vi "Protection and Rolling Counter Addon SysDef Example.vi"() -> (0 "error out":errorcluster)   [LabVIEW 2025]
uses:
  NationalInstruments.VeriStand.Internal
  NationalInstruments.VeriStand.SystemDefinitionAPI
  Protection and Counter Addon System Definition API.lvlib
panel:
  in  "Configuration (.dat)":path
  in  "error in (no error)":errorcluster
  out "Sysdef Path":path=path "C:/Users/Public/Documents/National Instruments/NI VeriStand 2013/DynamicallyCreatedProject/DynamicallyCreatedProject.nivssdf"
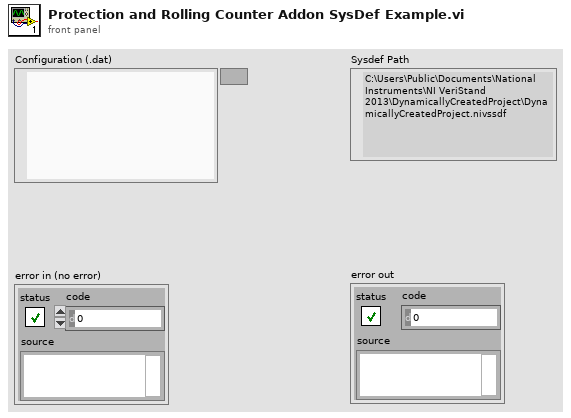
[diagram p1: front panel]
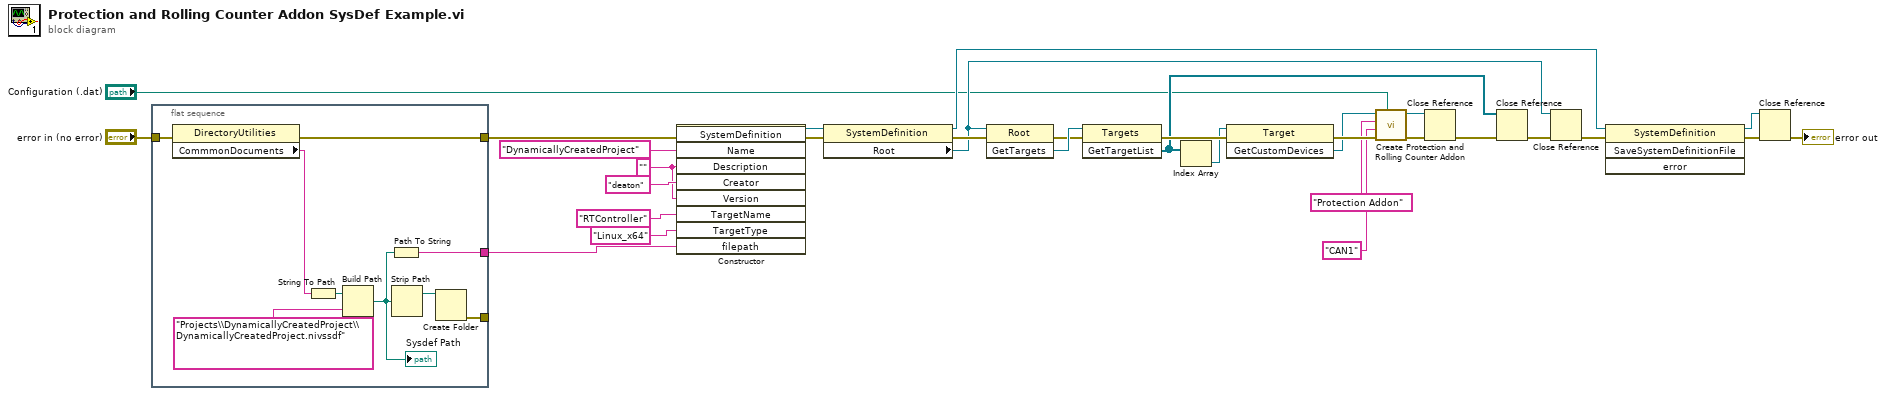
[diagram p0: block diagram]
diagram:
  w28 = "" ("Description")
  n1 = flat-sequence {
    tunnel: [w40] -> w27
    tunnel: "error in (no error)" -> [w34]
    tunnel: [w33] -> w7
    tunnel: [w32] -> _
    frame #0 {
      n2 = property class="DirectoryUtilities"(error in=w34) -> (error out=w33:errorcluster, "CommmonDocuments"=w38:string)  [unwired: 1 in, 1 out]
      n3 = String To Path(string=w38) -> (path=w37:path)
      n4 = Build Path(base path=w37, name or relative path="Projects\\DynamicallyCreatedProject\\DynamicallyCreatedProject.nivssdf") -> (appended path=w35:path)
      "Sysdef Path" <- w35
      n5 = Path To String(path=w35) -> (string=w40:string)
      n6 = Strip Path(path=w35) -> (stripped path=w39:path)  [unwired: 1 out]
      n7 = Create Folder(path (use dialog)=w39) -> (error out=w32:errorcluster)  [unwired: 2 in, 2 out]
    }
  }
  n8 = constructor class="SystemDefinition"(error in=w7, "Name"="DynamicallyCreatedProject", "Description"=w28, "Creator"="deaton", "Version"=w28, "TargetName"="RTController", "TargetType"="Linux_x64", "filepath"=w27) -> (reference out=w23:refnum<k24>, error out=w25:errorcluster)  [unwired: 2 in, 8 out]
  n9 = property class="SystemDefinition"(reference=w23, error in=w25) -> (reference out=w11:refnum<k24>, error out=w24:errorcluster, "Root"=w10:refnum<k24>)
  n10 = invoke class="Root" method="GetTargets"(reference=w10, error in=w24) -> (error out=w22:errorcluster, "GetTargets"=w26:refnum<k24>)  [unwired: 1 in, 1 out]
  n11 = invoke class="Targets" method="GetTargetList"(reference=w26, error in=w22) -> (error out=w20:errorcluster, "GetTargetList"=w9:refnum<k24>[])  [unwired: 1 in, 1 out]
  n12 = Index Array(array=w9) -> (element=w19:refnum<k24>)  [unwired: 1 in]
  n13 = invoke class="Target" method="GetCustomDevices"(reference=w19, error in=w20) -> (error out=w13:errorcluster, "GetCustomDevices"=w4:refnum<k24>)  [unwired: 1 in, 1 out]
  n14 = call "Create Protection and Rolling Counter Addon.vi"("Configuration (.dat)"="Configuration (.dat)", "error in (no error)"=w13, "Port"="CAN1", "Name"="Protection Addon", "Custom Devices Ref in"=w4) -> ("error out"=w6:errorcluster, "Custom Devices Ref"=w12:refnum<k24>)  [unwired: 5 in]
  n15 = Close Reference(reference=w12, error in (no error)=w6) -> (error out=w5:errorcluster)
  n16 = Close Reference(reference=w9, error in (no error)=w5) -> (error out=w17:errorcluster)
  n17 = Close Reference(reference=w10, error in (no error)=w17) -> (error out=w18:errorcluster)
  n18 = invoke class="SystemDefinition" method="SaveSystemDefinitionFile"(reference=w11, error in=w18) -> (reference out=w16:refnum<k24>, error out=w14:errorcluster)  [unwired: 2 in, 2 out]
  n19 = Close Reference(reference=w16, error in (no error)=w14) -> (error out=→"error out":errorcluster)
